vi "Fileout.vi"(8 "error in (no error)":errorcluster, 9 "Filepath":path, 10 "RecState":refnum<notifier>, 11 "Logging Queue":refnum<queue>) -> (0 "error out":errorcluster)   [LabVIEW 2018]
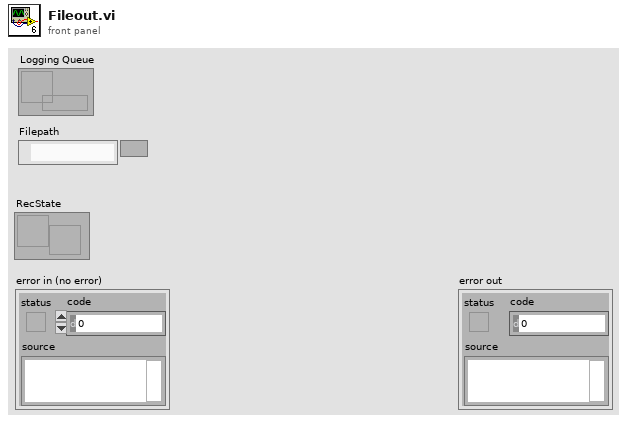
[diagram p1: front panel]
types:
  T1 = enum16{"Normal", "Overdrive", "Ready for Overdrive End", "Ready for new file", "New file"}
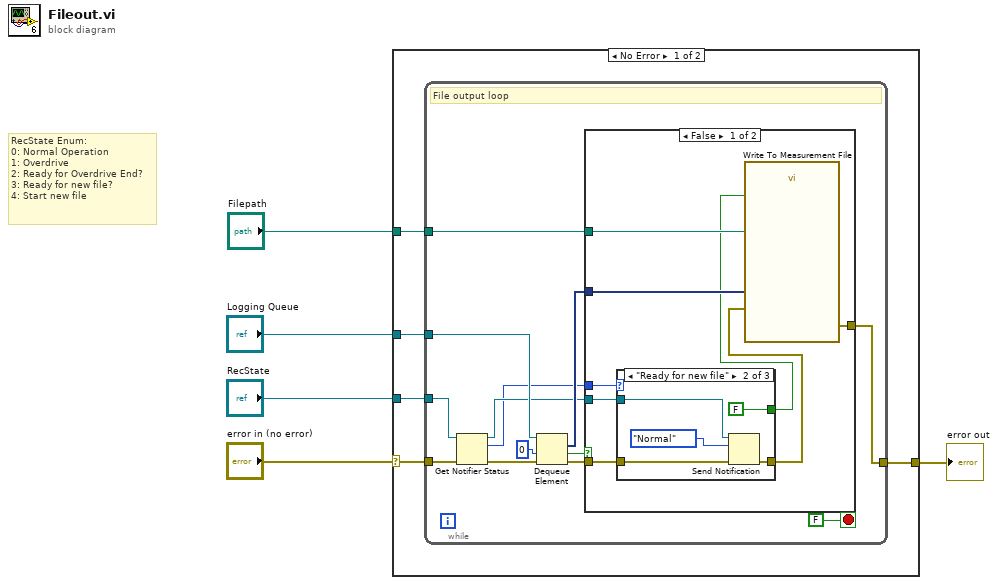
[diagram p0: block diagram]
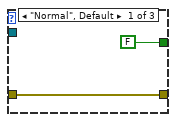
[diagram p2: hidden frame]
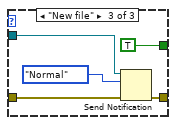
[diagram p3: hidden frame]
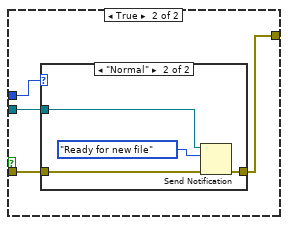
[diagram p4: hidden frame]
diagram:
  # "RecState Enum:\n0: Normal Operation\n1: Overdrive\n2: Ready for Overdrive End?\n3: Ready for new file?\n4: Start new file"
  n1 = case shown="No Error" "error in (no error)" {
    selector: "error in (no error)" -> [w9 w53]
    tunnel: [w6 w53] -> w2
    tunnel: "Logging Queue" -> [w10 _]
    tunnel: "Filepath" -> [w7 _]
    tunnel: "RecState" -> [w8 _]
    frame No Error {
      n2 = while {
        tunnel: w10 -> [w23]
        tunnel: w9 -> [w18]
        tunnel: w8 -> [w17]
        tunnel: w7 -> [w13]
        tunnel: [w12] -> w6
        stop <- FALSE stop-if-true
        # "File output loop"
        n3 = Get Notifier Status(notifier=w17, error in (no error)=w18) -> (notifier out=w15:refnum<notifier>, current notification=w14:T1, error out=w19:errorcluster)  [unwired: 2 out]
        n4 = Dequeue Element(queue=w23, timeout in ms (-1)=0, error in (no error)=w19) -> (element=w20:dynamicdata, timed out?=w21:bool, error out=w16:errorcluster)  [unwired: 1 out]
        n5 = case shown="False" w21 {
          tunnel: w14 -> [w31 w47]
          tunnel: w20 -> [w27 _]
          tunnel: w16 -> [w30 w46]
          tunnel: w15 -> [w29 w45]
          tunnel: w13 -> [w28 _]
          tunnel: [w24 w44] -> w12
          frame False {
            n6 = case shown="\"Ready for new file\"" w31 {
              tunnel: w30 -> [w33 w36 w43]
              tunnel: w29 -> [_ w37 w40]
              tunnel: [w33 w35 w42] -> w26
              tunnel: [FALSE FALSE TRUE] -> w25
              frame "Normal", Default {
              }
              frame "Ready for new file" {
                n7 = Send Notification(notification=T1."Normal" ("RecState"), notifier=w37, error in (no error)=w36) -> (error out=w35:errorcluster)  [unwired: 1 out]
              }
              frame "New file" {
                n8 = Send Notification(notification=T1."Normal" ("RecState"), notifier=w40, error in (no error)=w43) -> (error out=w42:errorcluster)  [unwired: 1 out]
              }
            }
            n9 = call "Write To Measurement File"("Signals"=w27, "new_file"=w25, "error in (no error)"=w26, "Filename"=w28) -> ("error out"=w24:errorcluster)  [unwired: 13 in, 2 out]
          }
          frame True {
            n10 = case shown="\"Normal\"" w47 {
              tunnel: [w48 w52] -> w44
              tunnel: w46 -> [w48 w51]
              tunnel: w45 -> [_ w50]
              frame Default {
              }
              frame "Normal" {
                n11 = Send Notification(notification=T1."Ready for new file" ("RecState"), notifier=w50, error in (no error)=w51) -> (error out=w52:errorcluster)  [unwired: 1 out]
              }
            }
          }
        }
      }
    }
    frame Error {
    }
  }
  "error out" <- w2
